vi "Fast mmWave Port Switching.vi"() -> ()   [LabVIEW 2019]
uses:
  <vilib>/Analysis/4window.llb/windowTd.ctl
  SubVIs/Low-level/TypeDefs/Resources.ctl
  <vilib>/userdefined/High Color/nirio_resource_hc.ctl
  SubVIs/Low-level/TypeDefs/Detected mmWave Adapters.ctl
  SubVIs/Low-level/TypeDefs/mmWave Adapter Information.ctl
  SubVIs/Low-level/TypeDefs/Front End Configuration.ctl
  SubVIs/Low-level/TypeDefs/Channel Configuration.ctl
  <instrlib>/niMmWave/ni3620/Config/v1/Host/Public/Typedefs/mmWave Port.ctl
  SubVIs/Low-level/TypeDefs/Hardware Configuration.ctl
  SubVIs/Low-level/TypeDefs/Direction.ctl
  SubVIs/Low-level/TypeDefs/Gain Setting.ctl
  <instrlib>/niMmWave/ni3620/Config/v1/FPGA/Public/Typedefs/TX1 RX1 Port.ctl
  SubVIs/mmWave HW Control/mmWave HW Control.lvlib
  <vilib>/Analysis/NI_AALPro.lvlib
  <instrlib>/niMmWave/ni3620/Config/v1/Host/niMmWave Config v1 Host.lvlib
panel:
  in  "indicators tab":T1(tab)=enum."Instructions"
  out "time domain":waveform(dbl)[](graph)
  out "frequency domain":cluster{"Ramp Pattern":dbl[], dbl[]}[](graph)
  in  "window":T2=8 items=["Rectangle"=0, "Hanning"=1, "Hamming"=2, "Blackman-Harris"=3, "Exact Blackman"=4, "Blackman"=5, "Flat Top"=6, "4 Term B-Harris "=7, "7 Term B-Harris"=8, "Low Sidelobe"=9, "Blackman Nuttall"=11, "Triangle"=30, "Bartlett-Hanning"=31, "Bohman"=32, "Parzen"=33, "Welch"=34, "Kaiser"=60, "Dolph-Chebyshev"=61, "Gaussian"=62]
  out "time domain power":waveform(dbl)[](graph)
  out "coerced device configuration [channel]":T3[](array[typedef]) {"Tx hardware configuration"."frequency (Hz)" format="%#_6p"; "Rx hardware configuration"."frequency (Hz)" format="%#_6p"}
  out "detected mmWave adapters [channel]":T6[](array[typedef]) {"detected mmWave adapters"."serial number" format="%.0x"}
  out "error out":errorcluster
  in  "stop":bool
  in  "controls tab":T9(tab)
  in  "option string":string="sample_rate=3.072G"
  in  "hardware resources [channel]":T10[](array[typedef])=[{"7902R (Tx)"="TxFpga0", "3610 (Tx)"="Dac0", "3620 (IF)"="IF0", "3630 (RX)"="Adc0", "7902R (Rx)"="RxFpga0"}]
  in  "hardware setup":T11
  in  "acquisition samples":u32=524288
  in  "tone frequency":dbl=500000000.0 format="%#_13p"
  in  "tone gain (dBFS)":dbl=-5.0 format="%#_13g"
  in  "device configuration [channel]":T3[](array[typedef])=[{"port select"=enum."IF Port", "Rx hardware configuration"={"gain (dB)"=20.0, "frequency (Hz)"=28500000000.0, "mmWave adapter"="mmWave0/0", "adapter active port"="RX1"}, "Tx hardware configuration"={"gain (dB)"=-20.0, "frequency (Hz)"=28500000000.0, "mmWave adapter"="mmWave0/0", "adapter active port"="TX1"}}] {"Tx hardware configuration"."frequency (Hz)" format="%#_6p"; "Rx hardware configuration"."frequency (Hz)" format="%#_6p"}
  in  "port list":T13[](array[typedef])=[enum."TX1/RX2", enum."RX1", enum."TX1/RX2", enum."RX1", enum."TX1/RX2"]
  in  "initial configuration":cluster{"scope":string, "gain setting":T14}[](array[cluster])=[{"scope"="rx", "gain setting"={"gain"=20.0, "port"=enum."RX1"}}, {"scope"="tx", "gain setting"={"gain"=-20.0, "port"=enum."TX1/RX2"}}]
  in  "port config trigger":string(combo)="PXI_Trig6"
  in  "port configurer scope":string(combo)="tx"
  in  "gain ranging enable controls":T15={"enable fine gain ranging"=FALSE, "enable coarse gain ranging"=FALSE, "enable port config"=TRUE}
  in  "dwell time (s)":dbl=5e-05 format="%#_13p"
  in  "update gain ranging settings":bool caption="update settings"
  # "Instructions:\n(1) Select device resources (Setup tab)\n(2) Select hardware setup (Setup tab)\n(3) Set device configuration\n         See datasheet for recommended gain settings\n          Warning: Incompatible gain settings may damage hardware.  \n                         Refer to datasheet for recommended gain settings.\n(4) Run this example\n\nNote: The Receiver and Transmitter must be connected (loopback) and the hardware configuration must be set\nto transceiver in order for channel equalization to occur.  When looping back at mmWave, be sure to \nconsult the datasheet to ensure sufficient path loss."
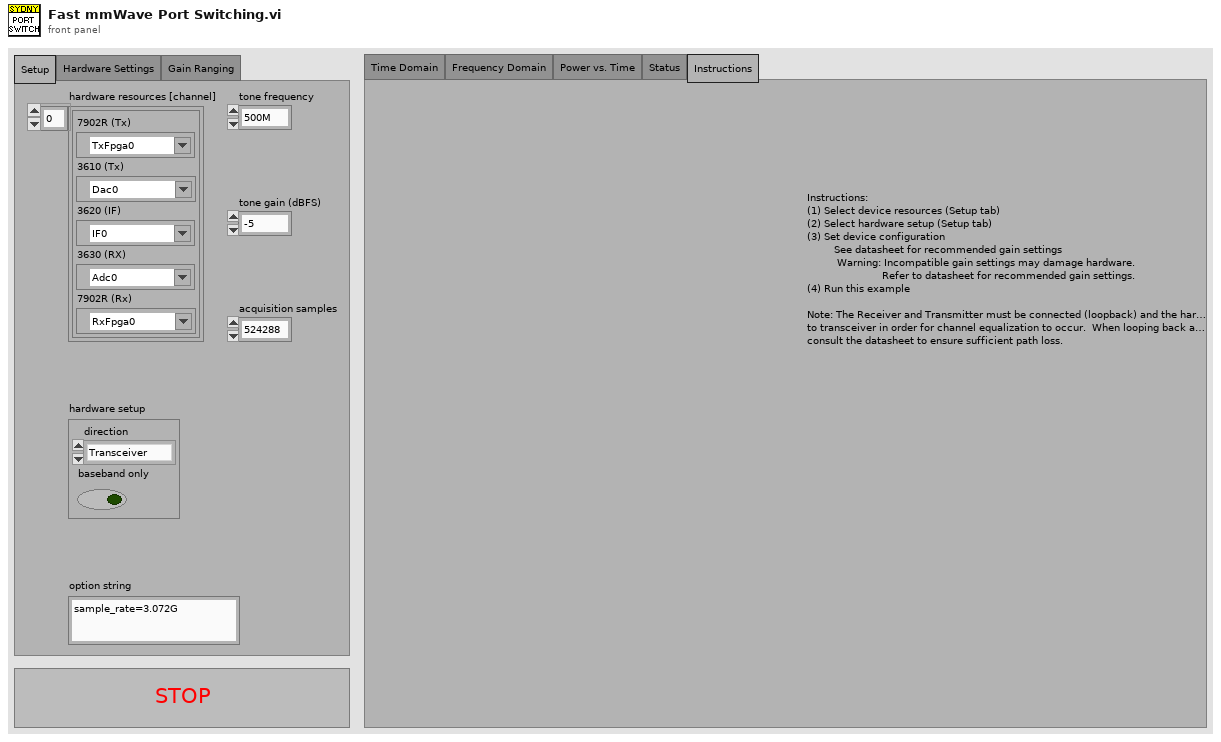
[diagram p1: front panel]
types:
  T1 = enum32{"Time Domain", "Frequency Domain", "Power vs. Time", "Status", "Instructions"}
  T2 = typedef "NI_AALPro.lvlib/windowTd.ctl" = u32
  T3 = typedef "Front End Configuration.ctl" = cluster{"port select":enum16{"IF Port", "Loopback", "Sync Port"}, "Rx hardware configuration":T4, "Tx hardware configuration":T4}
  T4 = typedef "Channel Configuration.ctl" = cluster{"gain (dB)":dbl, "frequency (Hz)":dbl, "mmWave adapter":string, "adapter active port":T5}
  T5 = typedef "niMmWave Config v1 Host.lvlib/mmWave Port.ctl" = string
  T6 = typedef "Detected mmWave Adapters.ctl" = cluster{"3620 resource name":T7, "detected mmWave adapters":T8[]}
  T7 = typedef "nirio_resource_hc.ctl" = tag
  T8 = typedef "mmWave Adapter Information.ctl" = cluster{"scope":string, "mmWave adapter type":string, "serial number":u64}
  T9 = enum32{"Setup", "Hardware Settings", "Gain Ranging"}
  T10 = typedef "Resources.ctl" = cluster{"7902R (Tx)":T7, "3610 (Tx)":refnum<visa-resource-name>, "3620 (IF)":T7, "3630 (RX)":refnum<visa-resource-name>, "7902R (Rx)":T7}
  T11 = typedef "Hardware Configuration.ctl" = cluster{"direction":T12, "baseband only":bool}
  T12 = typedef "Direction.ctl" = enum16{"Transceiver", "Receiver", "Transmitter"}
  T13 = typedef "TX1 RX1 Port.ctl" = enum8{"RX1", "TX1/RX2"}
  T14 = typedef "Gain Setting.ctl" = cluster{"gain":fxp<+/-,16,12>, "port":T13}
  T15 = cluster{"enable fine gain ranging":bool, "enable coarse gain ranging":bool, "enable port config":bool}
  T16 = typedef "Session.ctl" = cluster{"3620 session":refnum<queue>, "tx baseband session":T17, "rx baseband session":T25, "tx gain (dB)":dbl, "rx gain (dB)":dbl, "hardware configuration":T11, "gain ranging":T26[], "pxi trigger bus information":T27}
  T17 = typedef "Tx Baseband Session.ctl" = cluster{"3610 session":T18, "7902 reference":T24}
  T18 = typedef "ni3610_and_ni3630_Driver_Lib.lvlib/Main Settings.ctl" = cluster{"VISA resource name":refnum<visa-resource-name>, "Address Space":T19, "window_offset":u32, "register_addresses":T20, "required_MM_fpga_version":cluster{"signature":u32, "hardware":u32, "current revision":u32, "oldest revision":u32}, "CPLD Oldest Compat Version ":cluster{"hardware":u32, "CPLD firmware":u32}, "MM_FPGA_image_location":string, "is_init":bool, "card_type":T21, "DacLmkConfigFileName":string, "AdcLmkConfigFileName":string, "AdcConfigFileName":string, "DacConfigFileName_RevA":string, "DacConfigFileName_RevB":string, "Mulde hardware revision":u8, "bypass DAC PLL\n":bool, "IQ Card Revision":T22, "board capability":T23}
  T19 = typedef "VISA Register Access Address Space.ctl" = u16
  T20 = typedef "ni3610_and_ni3630_Driver_Lib.lvlib/Register Adresses.ctl" = cluster{"MM based Registers":cluster{"Revision":u32, "OldestCompatRev":u32, "signature":u32, "scratch":u32, "LedControl":u32, "BoardHwRev":u32, "BoardControl":u32, "ThermalStatus":u32, "BasebandStatus":u32, "BasebandControl":u32, "BasebandAuxSetup":u32, "BasebandAuxStatus":u32, "LmkSyncOutSetup":u32, " AdcSyncOutSetup":u32, " InjSyncOutSetup":u32, " PxiTrig0OutSetup":u32, " PxiTrig1OutSetup":u32, " PxiTrig2OutSetup":u32, " PxiTrig3OutSetup":u32, " PxiTrig4OutSetup":u32, " PxiTrig5OutSetup":u32, " PxiTrig6OutSetup":u32, " PxiTrig7OutSetup":u32}, "CPLD based Registers":cluster{"SlaveSignature":u32, "SlaveRevision":u32, "SlaveOldestCompatRev":u32, "SlaveScratch":u32, "SlaveSetup":u32, "SlaveStatus":u32, "IDacReg_offset":u32, "LMKRegGrp0_offset":u32, "QDacReg_offset":u32, "BrdTempSensorVal":u32, "TempSensorPowerDown":u32, "GPIOReg_offset":u32, "IAdcReg_offset":u32, "QAdcReg_offset":u32, "LMKRegGrp1_offset":u32, "QadcTempSensorVal":u32, "IadcTempSensorVal":u32, "RevisionReg":u32, "VcxoReg":u32, "CpldStatusReg":u32, "PowerReg":u32, "VBiasEnReg":u32, "ExtRefOeReg":u32, "QdacCtrlReg":u32, "QdacStatusReg":u32, "IdacCtrlReg":u32, "IdacStatusReg":u32, "QdacJtagIn":u32, "QdacJtagOut":u32, "IdacJtagIn":u32, "IdacJtagOut":u32, "IqDcSetupReg":u32, "QadcStatusReg":u32, "IadcStatusReg":u32, "BrdSetupReg":u32, "IqDcRevisionReg":u32, "PllStatusReg":u32, "EndpointScratchReg":u32, "AdcSyncCfgReg":u32, "IqCardOpampReg":u32}, "CPLD Register Offset":u32, "MM  Register Offset":u32, " PxiTrig0OutSetup":u32}
  T21 = typedef "ni3610_and_ni3630_Driver_Lib.lvlib/Base Card Type.ctl" = enum16{"unspecified", "ADC", "DAC"}
  T22 = typedef "ni3610_and_ni3630_Driver_Lib.lvlib/IQ Card Revision.ctl" = enum16{"RevA", "RevB", "RevC", "RevD"}
  T23 = typedef "ni3610_and_ni3630_Driver_Lib.lvlib/Board Capability.ctl" = cluster{"baseband sync":enum16{"no baseband sync", "baseband sync"}}
  T24 = typedef "Blank FPGA Reference.ctl" = refnum<k20>
  T25 = typedef "Rx Baseband Session.ctl" = cluster{"3630 session":T18, "7902 reference":T24}
  T26 = typedef "Gain Ranging.ctl" = cluster{"gain ranging active scope":string, "gain ranging stream session":refnum<k20>}
  T27 = typedef "PXI Trigger Bus Info.ctl" = cluster{"chassis resource name":refnum<visa-resource-name>, "7902R (TX)":i16, "3610 (TX)":i16, "3620 (IF)":i16, "3630 (RX)":i16, "7902R (RX)":i16}
  T28 = cluster{"frequency offset (Hz)":dbl[], "response":cdb[]}
  T29 = typedef "Constants.ctl" = cluster{"data clock rate (Hz)":dbl, "sample rate (Hz)":dbl, "sample rate selector string":string, "default tx bitfile path":path, "default rx bitfile path":path, "default proc bitfile path":path}
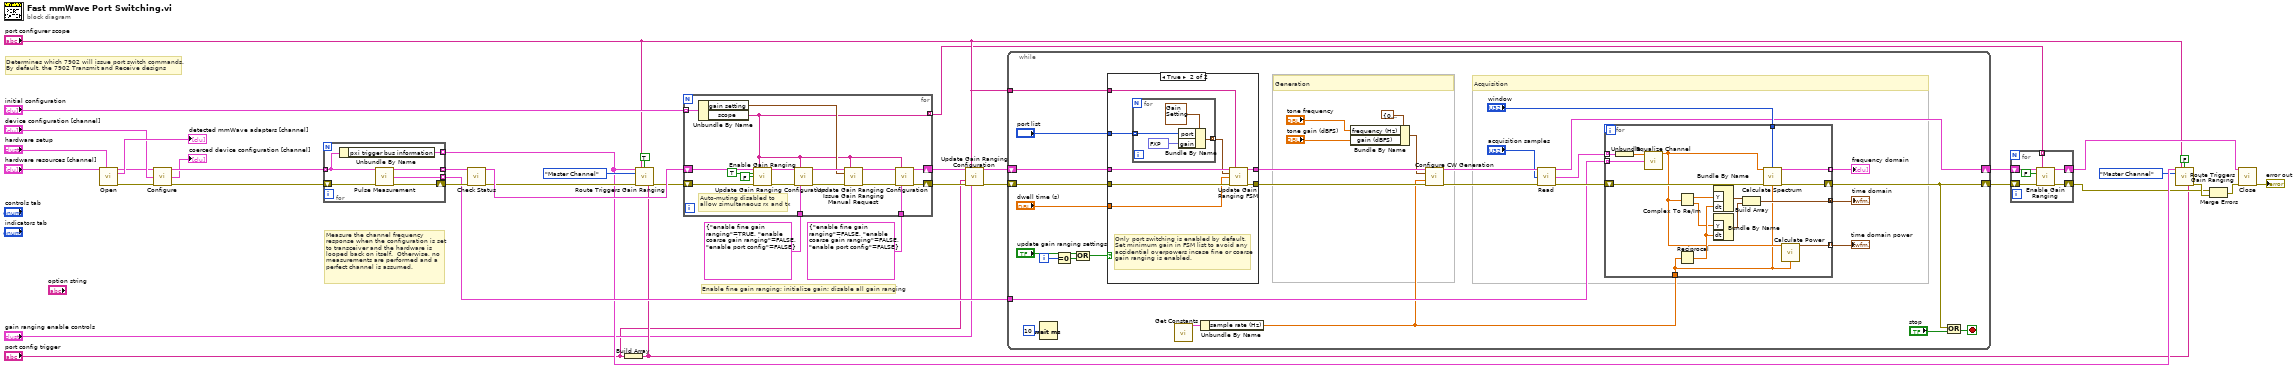
[diagram p0: block diagram]
diagram:
  # "Determines which 7902 will issue port switch commands.\nBy default, the 7902 Transmit and Receive designs"
  # "Enable fine gain ranging; initialize gain; disable all gain ranging"
  # "Measure the channel frequency\nresponse when the configuration is set\nto transceiver and the hardware is \nlooped back on itself.  Otherwise, no\nmeasurements are performed and a\nperfect channel is assumed."
  n1 = call "Open.vi"("resources"="hardware resources [channel]", "hardware configuration"="hardware setup") -> ("session out"=w31:T16[], "detected mmWave adapters"=→"detected mmWave adapters [channel]":T6[], "error out"=w30:errorcluster)  [unwired: 11 in]
  n2 = call "Configure.vi"("session in"=w31, "device configuration [channel]"="device configuration [channel]", "error in"=w30) -> ("session out"=w34:T16[], "coerced device configuration [channel]"=→"coerced device configuration [channel]":T3[], "error out"=w33:errorcluster)  [unwired: 10 in]
  n3 = for {
    shift-right: [w44] -> w36
    shift-left: w33 -> [w42]
    tunnel: w34 -> [w41] mode=indexing
    tunnel: [w45] -> w35 mode=indexing
    tunnel: [w43] -> w32 mode=indexing
    tunnel: [w40] -> w18 mode=indexing
    n4 = Unbundle By Name(w41) -> ("pxi trigger bus information"=w40:T27)
    n5 = call "Pulse Measurement.vi"("session"=w41, "error in"=w42) -> ("session out"=w45:T16, "channel"=w43:T28, "error out"=w44:errorcluster)  [unwired: 11 in]
  }
  n6 = call "Check Status.vi"("session in"=w35, "error in"=w36) -> ("session out"=w23:T16[], "error out"=w19:errorcluster)  [unwired: 9 in, 3 out]
  n7 = Build Array("port config trigger") -> (w12:string[])
  n8 = call "Route Triggers Gain Ranging.vi"("pxi trigger bus configuration [channel]"=w18, "scope"="port configurer scope", "map(T)/unmap(F)"=TRUE, "routing mode"=enum16{"Master Channel", "Independent Channels"}."Master Channel" ("Routing Mode"), "error in"=w19, "mmWave port config PXI trigger [channel]"=w12) -> ("error out"=w22:errorcluster)  [unwired: 9 in]
  n9 = for {
    shift-right: [w52] -> w6
    shift-left: w23 -> [w62]
    shift-right: [w51] -> w8
    shift-left: w22 -> [w61]
    tunnel: T15 {"enable fine gain ranging"=TRUE, "enable coarse gain ranging"=FALSE, "enable port config"=FALSE} ("enables") -> [w57]
    tunnel: T15 {"enable fine gain ranging"=FALSE, "enable coarse gain ranging"=FALSE, "enable port config"=FALSE} ("enables") -> [w50]
    tunnel: "initial configuration" -> [w49] mode=indexing
    tunnel: [w47] -> w1 mode=indexing
    # "Auto-muting disabled to\nallow simultaneous rx and tx"
    n10 = Unbundle By Name(w49) -> ("gain setting"=w48:T14, "scope"=w47:string)
    n11 = call "Enable Gain Ranging.vi"("session in"=w62, "scope"=w47, "enable"=TRUE, "TRx LO auto-muting"=FALSE, "error in"=w61) -> ("session out"=w58:T16[], "error out"=w59:errorcluster)  [unwired: 9 in]
    n12 = call "Update Gain Ranging Configuration.vi"("session in"=w58, "scope"=w47, "error in"=w59, "enables"=w57) -> ("session out"=w55:T16[], "error out"=w56:errorcluster)  [unwired: 9 in, 1 out]
    n13 = call "Issue Gain Ranging Manual Request.vi"("session in"=w55, "scope"=w47, "gain ranging manual request"=w48, "error in"=w56) -> ("session out"=w53:T16[], "error out"=w54:errorcluster)  [unwired: 10 in]
    n14 = call "Update Gain Ranging Configuration.vi"("session in"=w53, "scope"=w47, "error in"=w54, "enables"=w50) -> ("session out"=w52:T16[], "error out"=w51:errorcluster)  [unwired: 9 in, 1 out]
  }
  n15 = call "Update Gain Ranging Configuration.vi"("session in"=w6, "scope"="port configurer scope", "mmWave port config PXI trigger"="port config trigger", "error in"=w8, "enables"="gain ranging enable controls") -> ("session out"=w5:T16[], "error out"=w7:errorcluster)  [unwired: 8 in, 1 out]
  n16 = while {
    shift-right: [w89] -> w29
    shift-left: w7 -> [w82]
    shift-right: [w88] -> w28
    shift-left: w5 -> [w83]
    tunnel: w32 -> [w86]
    tunnel: "port configurer scope" -> [w66]
    i -> [w80]
    stop <- w95 stop-if-true
    # "Generation"
    # "Acquisition"
    n17 = Wait (ms)(milliseconds to wait=u32 10) -> ()  [unwired: 1 out]
    n18 = Wait (ms)(milliseconds to wait=u32 10) -> ()  [unwired: 1 out]
    n19 = Equal To 0?(x=w80) -> (x = 0?=w77:bool)
    n20 = Compound Arithmetic op=OR("update gain ranging settings", w77) -> (w79:bool)
    n21 = case shown="True" w79 {
      tunnel: w83 -> [w97 w104]
      tunnel: w82 -> [w96 w105]
      tunnel: [w97 w103] -> w76
      tunnel: [w96 w102] -> w74
      tunnel: "dwell time (s)" -> [_ w100]
      tunnel: w66 -> [_ w101]
      tunnel: "port list" -> [_ w98]
      frame False {
      }
      frame True {
        # "Only port switching is enabled by default.\nSet minimum gain in FSM list to avoid any\naccidential overpowers incase fine or coarse\ngain ranging is enabled."
        n22 = for {
          tunnel: [w108] -> w99 mode=indexing
          tunnel: w98 -> [w107] mode=indexing
          n23 = Bundle By Name(cluster=T14 {"gain"=0.0, "port"=enum."RX1"} ("gain setting"), "port"=w107, "gain"=fxp<+/-,16,12> -2048.0) -> (w108:T14)
        }
        n24 = call "Update Gain Ranging FSM.vi"("session in"=w104, "scope"=w101, "gain setting list"=w99, "gain dwell time (s)"=w100, "error in"=w105) -> ("session out"=w103:T16[], "error out"=w102:errorcluster)  [unwired: 9 in]
      }
    }
    n25 = call "Get Constants.vi"() -> ("constants"=w69:T29)  [unwired: 15 in]
    n26 = Unbundle By Name(w69) -> ("sample rate (Hz)"=w67:dbl)
    n27 = Bundle By Name(cluster=cluster{"frequency (Hz)":dbl, "gain (dBFS)":dbl} {"frequency (Hz)"=0.0, "gain (dBFS)"=-3.0103} ("tone 1"), "frequency (Hz)"="tone frequency", "gain (dBFS)"="tone gain (dBFS)") -> (w70:cluster{"frequency (Hz)":dbl, "gain (dBFS)":dbl})
    n28 = call "Configure CW Generation.vi"("session in"=w76, "tone 1"=w70, "sample rate"=w67, "error in"=w74) -> ("session out"=w73:T16[], "error out"=w72:errorcluster)  [unwired: 10 in]
    n29 = call "Read.vi"("session in"=w73, "number of samples"="acquisition samples", "error in"=w72) -> ("session out"=w88:T16[], "data [channel]"=w64:cluster{"data":cdb[]}[], "error out"=w87:errorcluster)  [unwired: 10 in]
    n30 = for {
      tunnel: [w125] -> w85 mode=concatenating
      tunnel: [w124] -> w91 mode=indexing
      tunnel: "window" -> [w123]
      shift-right: [w122] -> w89
      shift-left: w87 -> [w121]
      tunnel: w64 -> [w119] mode=indexing
      tunnel: w86 -> [w118] mode=indexing
      tunnel: [w117] -> w84 mode=indexing
      tunnel: w67 -> [w110]
      n31 = Unbundle(w119) -> ("data"=w120:cdb[])
      n32 = call "Equalize Channel.vi"("input data"=w120, "channel"=w118) -> ("output data"=w113:cdb[])  [unwired: 13 in]
      n33 = Reciprocal(x=w110) -> (1/x=w115:dbl)
      n34 = Complex To Re/Im(x + iy=w113) -> (x=w116:dbl[], y=w114:dbl[])
      n35 = Bundle By Name("Y"=w116, "dt"=w115) -> (w112:waveform(dbl))  [unwired: 1 in]
      n36 = Bundle By Name("Y"=w114, "dt"=w115) -> (w111:waveform(dbl))  [unwired: 1 in]
      n37 = Build Array(w112, w111) -> (w125:waveform(dbl)[])
      n38 = call "Calculate Spectrum.vi"("input data"=w113, "window"=w123, "error in"=w121, "IQ rate"=w110) -> ("spectrum output"=w124:cluster{"Ramp Pattern":dbl[], dbl[]}, "error out"=w122:errorcluster)  [unwired: 10 in]
      n39 = call "Calculate Power.vi"("input data"=w113, "IQ rate"=w110) -> ("time domain power output"=w117:waveform(dbl))  [unwired: 13 in]
    }
    "time domain" <- w85
    "frequency domain" <- w91
    "time domain power" <- w84
    n40 = Compound Arithmetic op=OR(w89, "stop") -> (w95:bool)
  }
  n41 = for {
    tunnel: w1 -> [w126] mode=indexing
    shift-right: [w127] -> w13
    shift-left: w29 -> [w131]
    shift-right: [w129] -> w27
    shift-left: w28 -> [w130]
    n42 = call "Enable Gain Ranging.vi"("session in"=w130, "scope"=w126, "enable"=FALSE, "error in"=w131) -> ("session out"=w129:T16[], "error out"=w127:errorcluster)  [unwired: 10 in]
  }
  n43 = call "Route Triggers Gain Ranging.vi"("pxi trigger bus configuration [channel]"=w18, "scope"="port configurer scope", "map(T)/unmap(F)"=FALSE, "routing mode"=enum16{"Master Channel", "Independent Channels"}."Master Channel" ("Routing Mode"), "mmWave port config PXI trigger [channel]"=w12) -> ("error out"=w17:errorcluster)  [unwired: 10 in]
  n44 = Merge Errors(w13, w17) -> (w16:errorcluster)
  n45 = call "Close.vi"("session"=w27, "error in"=w16) -> ("error out"=→"error out":errorcluster)  [unwired: 13 in]
